vi "Convert ILC Voltage to Force.vi"(8 "error in (no error)":errorcluster, 10 "Voltage":dbl[unit], 11 "Model in":refnum<class "Model.lvclass">) -> (0 "error out":errorcluster, 2 "Force":dbl[unit], 3 "Model out":refnum<class "Model.lvclass">)   [LabVIEW 2015, in "Model.lvclass"]
uses:
  Model.lvclass
  Model.lvclass/Model.ctl
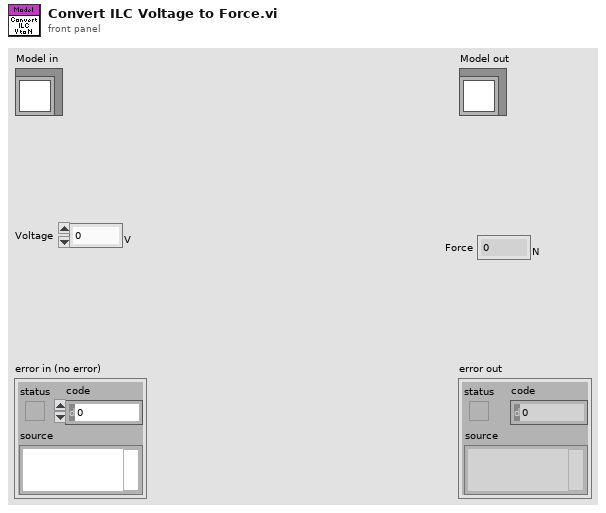
[diagram p1: front panel]
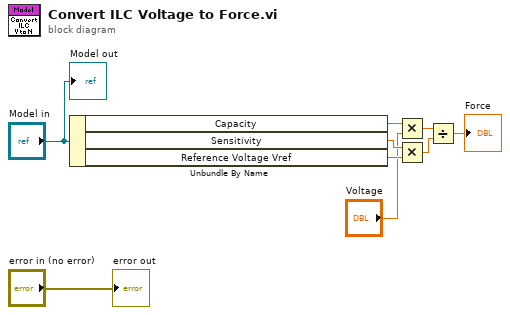
[diagram p0: block diagram]
diagram:
  n1 = Unbundle By Name("Model in") -> ("Capacity"=w6:dbl[unit], "Sensitivity"=w8:dbl[unit], "Reference Voltage Vref"=w7:dbl[unit])
  n2 = Multiply(x=w6, y="Voltage") -> (x*y=w4:dbl[unit])
  n3 = Multiply(x=w8, y=w7) -> (x*y=w3:dbl[unit])
  n4 = Divide(x=w4, y=w3) -> (x/y=→"Force":dbl[unit])
  "error out" <- "error in (no error)"
  "Model out" <- "Model in"
